vi "FeedbackDecode_UpdatePresetsTable.vi"(2 "StimClustIn":T1={"ParamsTable"=[], "Sel"=[], "Stim"=FALSE, "StimMode"=enum."Off", "StimStep"=[enum."1uA", enum."1uA", enum."Off"], "Jitter"=FALSE, "Pulse"=FALSE, "BFreq"=0.0, "BAmp"=0.0, "UEAArray"=[], "AdjClust"={"Add"=FALSE, "Sub"=FALSE, "Val"=[1.0, 100.0, 0.2, 500.0, 0.0], "B"=[FALSE, FALSE, FALSE, FALSE, FALSE], "Inc+"=["x+1", "x+10", "x+0.1", "x+10", "x+10"], "Set"=FALSE, "LoadTable"=FALSE, "SaveTable"=FALSE, "ClearTable"=FALSE, "DeleteSel"=FALSE, "Inc-"=["x-1", "x-10", "x-0.1", "x-10", "x-10"]}, "PresetTable"=[], "SelPreset"=[], "SortClust"={"Region"=FALSE, "Receptor"=FALSE, "Electrode"=FALSE, "Min Amp"=FALSE, "Max Amp"=FALSE, "Min Freq"=FALSE, "Max Freq"=FALSE, "Duration"=FALSE}, "SelSort"={"Sel"=FALSE}, "PresetClust"={"Load"=FALSE, "Clear"=FALSE, "Save"=FALSE, "Del"=FALSE}, "RespClust"={"RespType"=enum."Sensor Map", "OpenResp"=FALSE}, "AmpLimit"=0.0, "FreqLimit"=0.0, "DurLimit"=0.0, "Wait Period"=0.0, "Train Period"=0.0} {"Train Period" min=0.0 max=100.0 step=0.1; "Wait Period" min=0.0 max=100.0 step=0.1; "DurLimit" min=0.0 max=1.0 step=0.01; "FreqLimit" min=0.0 max=500.0 step=1.0; "AmpLimit" min=0.0 max=100.0 step=1.0; "BAmp" min=0.0 max=100.0 step=1.0; "BFreq" min=0.0 max=100.0 step=1.0}) -> (0 "StimClustOut":T1={"ParamsTable"=[], "Sel"=[], "Stim"=FALSE, "StimMode"=enum."Off", "StimStep"=[enum."1uA", enum."1uA", enum."Off"], "Jitter"=FALSE, "Pulse"=FALSE, "BFreq"=0.0, "BAmp"=0.0, "UEAArray"=[], "AdjClust"={"Add"=FALSE, "Sub"=FALSE, "Val"=[1.0, 100.0, 0.2, 500.0, 0.0], "B"=[FALSE, FALSE, FALSE, FALSE, FALSE], "Inc+"=["x+1", "x+10", "x+0.1", "x+10", "x+10"], "Set"=FALSE, "LoadTable"=FALSE, "SaveTable"=FALSE, "ClearTable"=FALSE, "DeleteSel"=FALSE, "Inc-"=["x-1", "x-10", "x-0.1", "x-10", "x-10"]}, "PresetTable"=[], "SelPreset"=[], "SortClust"={"Region"=FALSE, "Receptor"=FALSE, "Electrode"=FALSE, "Min Amp"=FALSE, "Max Amp"=FALSE, "Min Freq"=FALSE, "Max Freq"=FALSE, "Duration"=FALSE}, "SelSort"={"Sel"=FALSE}, "PresetClust"={"Load"=FALSE, "Clear"=FALSE, "Save"=FALSE, "Del"=FALSE}, "RespClust"={"RespType"=enum."Sensor Map", "OpenResp"=FALSE}, "AmpLimit"=0.0, "FreqLimit"=0.0, "DurLimit"=0.0, "Wait Period"=0.0, "Train Period"=0.0} {"Train Period" min=0.0 max=100.0 step=0.1; "Wait Period" min=0.0 max=100.0 step=0.1; "DurLimit" min=0.0 max=1.0 step=0.01; "FreqLimit" min=0.0 max=500.0 step=1.0; "AmpLimit" min=0.0 max=100.0 step=1.0; "BAmp" min=0.0 max=100.0 step=1.0; "BFreq" min=0.0 max=100.0 step=1.0})   [LabVIEW 2020]
uses:
  FeedbackDecode_EncodeClust.ctl
  <vilib>/regexp/Match Regular Expression.xnode
panel:
  # "Value"
  # "Inc-"
  # "Inc+"
  # "Min Amp"
  # "Max Amp"
  # "Min Freq"
  # "Max Freq"
  # "Duration"
  # "Value"
  # "Inc-"
  # "Inc+"
  # "Min Amp"
  # "Max Amp"
  # "Min Freq"
  # "Max Freq"
  # "Duration"
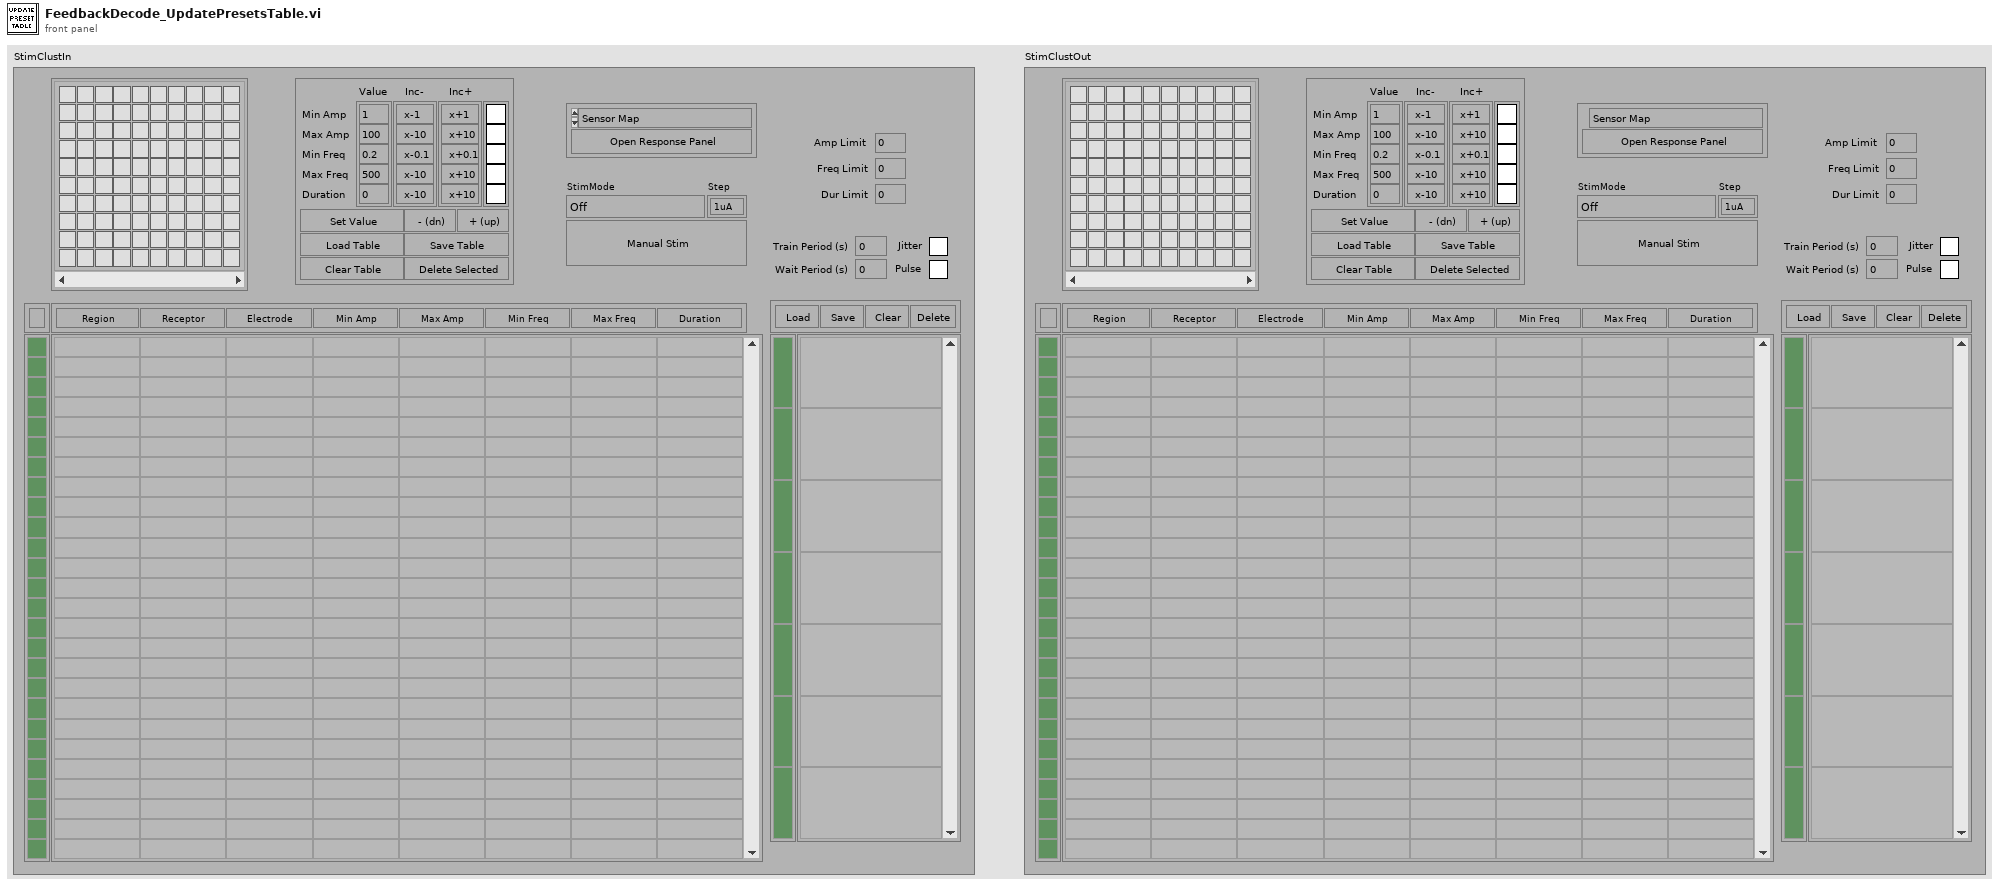
[diagram p1: front panel]
types:
  T1 = typedef "FeedbackDecode_EncodeClust.ctl" = cluster{"ParamsTable":string[][], "Sel":bool[], "Stim":bool, "StimMode":enum16{"Off", "Manual", "MSMS", "VRE", "3DHand", "DEKA", "Analog(DEKA)"}, "StimStep":enum16{"Off", "1uA", "2uA", "5uA", "10uA", "20uA", "30uA"}[], "Jitter":bool, "Pulse":bool, "BFreq":dbl, "BAmp":dbl, "UEAArray":cluster{"Boolean 1":bool, "Boolean 2":bool, "Boolean 3":bool, "Boolean 4":bool, "Boolean 5":bool, "Boolean 6":bool, "Boolean 7":bool, "Boolean 8":bool, "Boolean 9":bool, "Boolean 10":bool, "Boolean 11":bool, "Boolean 12":bool, "Boolean 13":bool, "Boolean 14":bool, "Boolean 15":bool, "Boolean 16":bool, "Boolean 17":bool, "Boolean 18":bool, "Boolean 19":bool, "Boolean 20":bool, "Boolean 21":bool, "Boolean 22":bool, "Boolean 23":bool, "Boolean 24":bool, "Boolean 25":bool, "Boolean 26":bool, "Boolean 27":bool, "Boolean 28":bool, "Boolean 29":bool, "Boolean 30":bool, "Boolean 31":bool, "Boolean 32":bool, "Boolean 33":bool, "Boolean 34":bool, "Boolean 35":bool, "Boolean 36":bool, "Boolean 37":bool, "Boolean 38":bool, "Boolean 39":bool, "Boolean 40":bool, "Boolean 41":bool, "Boolean 42":bool, "Boolean 43":bool, "Boolean 44":bool, "Boolean 45":bool, "Boolean 46":bool, "Boolean 47":bool, "Boolean 48":bool, "Boolean 49":bool, "Boolean 50":bool, "Boolean 51":bool, "Boolean 52":bool, "Boolean 53":bool, "Boolean 54":bool, "Boolean 55":bool, "Boolean 56":bool, "Boolean 57":bool, "Boolean 58":bool, "Boolean 59":bool, "Boolean 60":bool, "Boolean 61":bool, "Boolean 62":bool, "Boolean 63":bool, "Boolean 64":bool, "Boolean 65":bool, "Boolean 66":bool, "Boolean 67":bool, "Boolean 68":bool, "Boolean 69":bool, "Boolean 70":bool, "Boolean 71":bool, "Boolean 72":bool, "Boolean 73":bool, "Boolean 74":bool, "Boolean 75":bool, "Boolean 76":bool, "Boolean 77":bool, "Boolean 78":bool, "Boolean 79":bool, "Boolean 80":bool, "Boolean 81":bool, "Boolean 82":bool, "Boolean 83":bool, "Boolean 84":bool, "Boolean 85":bool, "Boolean 86":bool, "Boolean 87":bool, "Boolean 88":bool, "Boolean 89":bool, "Boolean 90":bool, "Boolean 91":bool, "Boolean 92":bool, "Boolean 93":bool, "Boolean 94":bool, "Boolean 95":bool, "Boolean 96":bool, "Boolean 97":bool, "Boolean 98":bool, "Boolean 99":bool, "Boolean 100":bool}[], "AdjClust":cluster{"Add":bool, "Sub":bool, "Val":dbl[], "B":bool[], "Inc+":string[], "Set":bool, "LoadTable":bool, "SaveTable":bool, "ClearTable":bool, "DeleteSel":bool, "Inc-":string[]}, "PresetTable":string[][], "SelPreset":bool[], "SortClust":cluster{"Region":bool, "Receptor":bool, "Electrode":bool, "Min Amp":bool, "Max Amp":bool, "Min Freq":bool, "Max Freq":bool, "Duration":bool}, "SelSort":cluster{"Sel":bool}, "PresetClust":cluster{"Load":bool, "Clear":bool, "Save":bool, "Del":bool}, "RespClust":cluster{"RespType":enum16{"Sensor Map", "Full Map"}, "OpenResp":bool}, "AmpLimit":dbl, "FreqLimit":dbl, "DurLimit":dbl, "Wait Period":dbl, "Train Period":dbl}
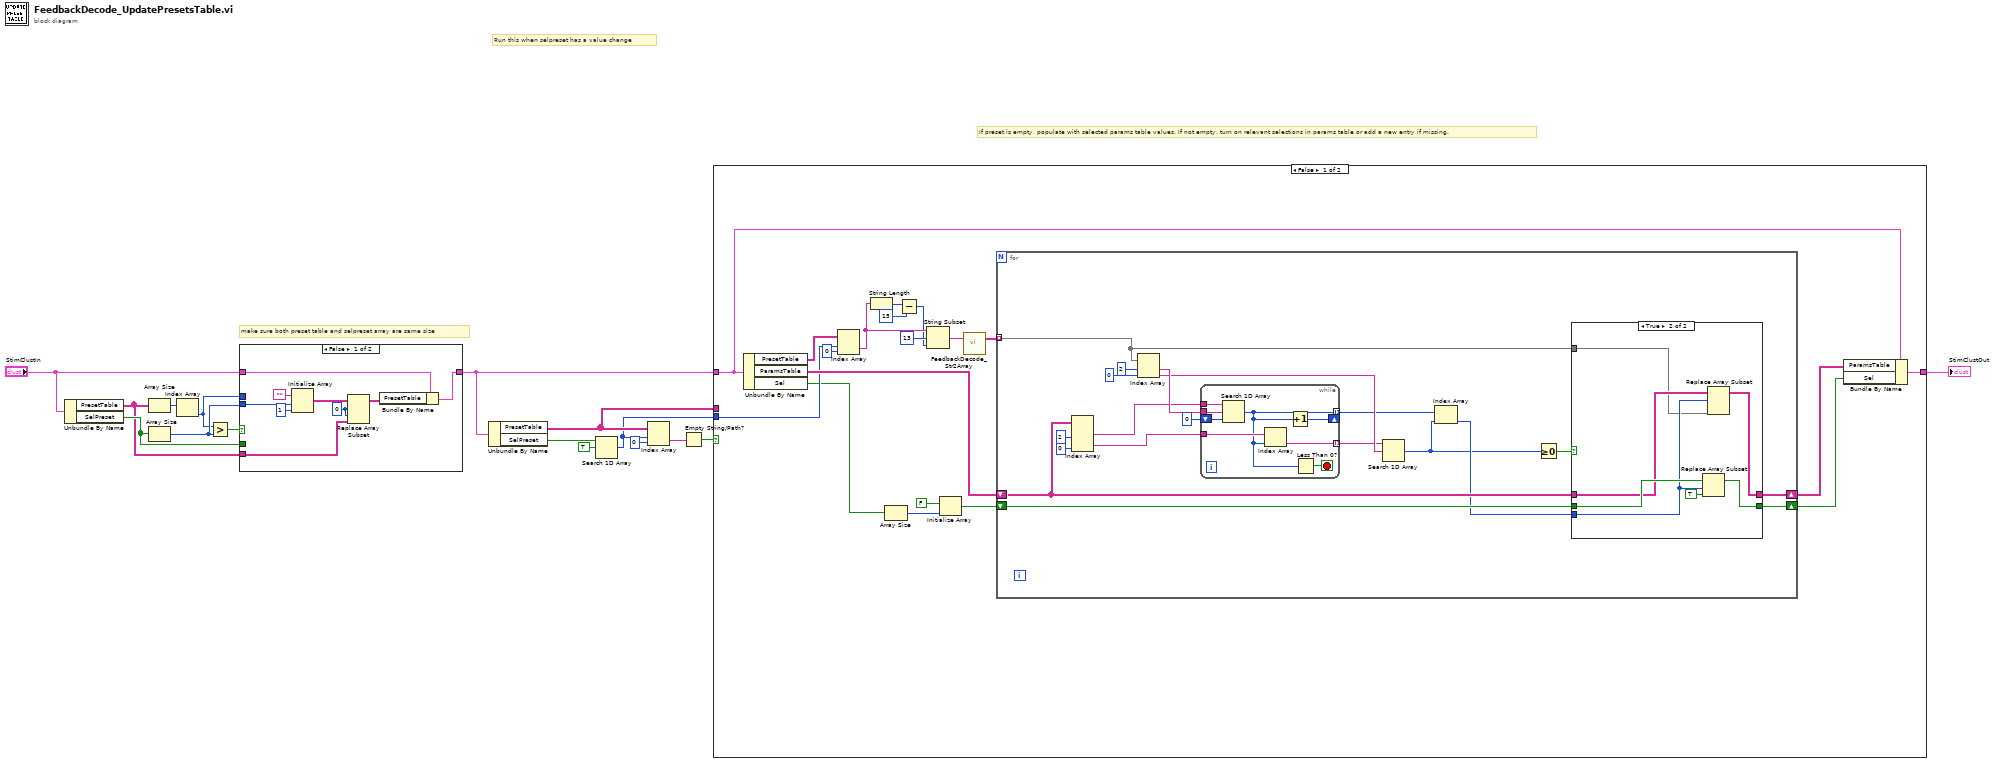
[diagram p0: block diagram]
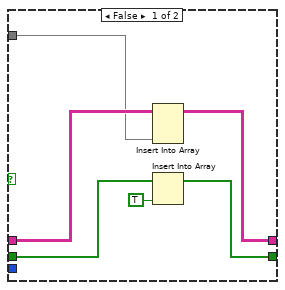
[diagram p2: hidden frame]
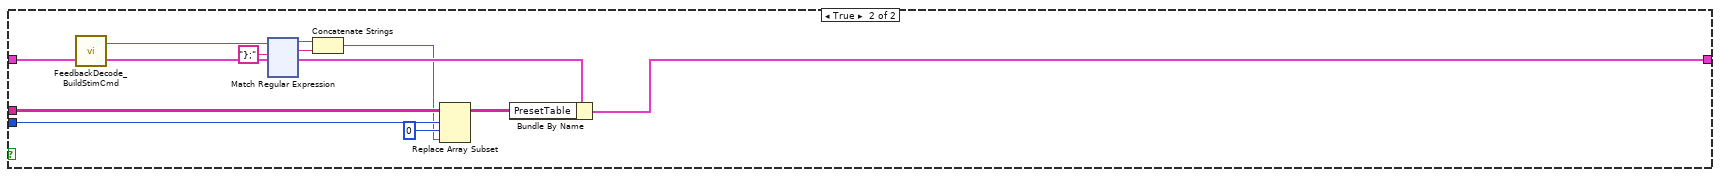
[diagram p3: hidden frame]
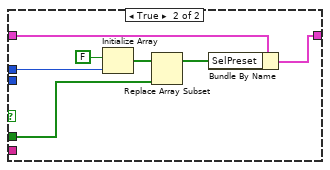
[diagram p4: hidden frame]
diagram:
  # "Run this when selpreset has a value change"
  # "If preset is empty, populate with selected params table values. If not empty, turn on relevant selections in params table or add a new entry if missing."
  # "make sure both preset table and selpreset array are same size"
  n1 = Unbundle By Name("StimClustIn") -> ("PresetTable"=w10:string[][], "SelPreset"=w14:bool[])
  n2 = Array Size(array=w10) -> (size(s)=w12:i32[])
  n3 = Array Size(array=w14) -> (size(s)=w16:i32)
  n4 = Index Array(array=w12) -> (element=w15:i32)  [unwired: 1 in]
  n5 = Greater?(x=w15, y=w16) -> (0:w13:bool)
  n6 = case shown="False" w13 {
    tunnel: "StimClustIn" -> [w23 w32]
    tunnel: [w22 w30] -> w4
    tunnel: w14 -> [_ w26]
    tunnel: w15 -> [_ w28]
    tunnel: w10 -> [w25 _]
    tunnel: w16 -> [w20 _]
    frame False {
      w24 = 0 ("index (row)")
      n7 = Initialize Array("", w20, 1 ("dimension size")) -> (w17:string[][])
      n8 = Replace Array Subset(array=w17, new element=w25, index (row)=w24, index (col)=w24) -> (w21:string[][])
      n9 = Bundle By Name(cluster=w23, "PresetTable"=w21) -> (w22:T1)
    }
    frame True {
      n10 = Initialize Array(FALSE ("new element/subarray"), w28) -> (w27:bool[])
      n11 = Replace Array Subset(array=w27, new element=w26) -> (w31:bool[])  [unwired: 1 in]
      n12 = Bundle By Name(cluster=w32, "SelPreset"=w31) -> (w30:T1)
    }
  }
  n13 = Unbundle By Name(w4) -> ("PresetTable"=w2:string[][], "SelPreset"=w9:bool[])
  n14 = Search 1D Array(1D array=w9, element=TRUE) -> (index of element=w1:i32)  [unwired: 1 in]
  n15 = Index Array(array=w2, index (row)=w1, index (col)=0 ("disabled index (col)")) -> (element=w7:string)
  n16 = Empty String/Path?(string/path=w7) -> (empty?=w6:bool)
  n17 = case shown="False" w6 {
    tunnel: w4 -> [w47 w97]
    tunnel: [w48 w98] -> w3
    tunnel: w2 -> [_ w102]
    tunnel: w1 -> [w45 w101]
    frame False {
      n18 = Unbundle By Name(w47) -> ("PresetTable"=w46:string[][], "ParamsTable"=w49:string[][], "Sel"=w37:bool[])
      n19 = Index Array(array=w46, index (row)=w45, index (col)=0 ("disabled index (col)")) -> (element=w40:string)
      n20 = String Length(string=w40) -> (length=w42:i32)
      n21 = Array Size(array=w37) -> (size(s)=w36:i32)
      n22 = Subtract(x=w42, y=15) -> (x-y=w38:i32)
      n23 = String Subset(string=w40, offset (0)=13, length (rest)=w38) -> (substring=w39:string)
      n24 = Initialize Array(FALSE, w36) -> (w34:bool[])
      n25 = call "FeedbackDecode_Str2Array.vi"("StringIn"=w39) -> ("StrArrayOut"=w33:string[][])  [unwired: 1 in, 1 out]
      n26 = for {
        shift-right: [w69] -> w51
        shift-left: w34 -> [w70]
        shift-right: [w67] -> w50
        shift-left: w49 -> [w68]
        tunnel: w33 -> [w53] mode=indexing
        n27 = Index Array(array=w68, index (col) #1=2 ("disabled index (col)"), index (col) #2=0 ("index (col)")) -> (element #1=w61:string[], element #2=w60:string[])  [unwired: 2 in]
        n28 = Index Array(array=w53, index #1=2 ("index"), index #2=0 ("index")) -> (element #1=w65:string, element #2=w59:string)
        n29 = while {
          tunnel: w61 -> [w78]
          tunnel: w65 -> [w77]
          shift-right: [w71] -> _
          shift-left: 0 ("disabled index (col)") -> [w76]
          tunnel: w60 -> [w75]
          tunnel: [w74] -> w58 mode=indexing
          tunnel: [w72] -> w57 mode=indexing
          stop <- w73 stop-if-true
          n30 = Search 1D Array(1D array=w78, element=w77, start index (0)=w76) -> (index of element=w72:i32)
          n31 = Index Array(array=w75, index=w72) -> (element=w74:string)
          n32 = Increment(x=w72) -> (x+1=w71:i32)
          n33 = Less Than 0?(x=w72) -> (x < 0?=w73:bool)
        }
        n34 = Search 1D Array(1D array=w58, element=w59) -> (index of element=w55:i32)  [unwired: 1 in]
        n35 = Index Array(array=w57, index=w55) -> (element=w56:i32)
        n36 = Greater Or Equal To 0?(x=w55) -> (x >= 0?=w54:bool)
        n37 = case shown="True" w54 {
          tunnel: w56 -> [_ w86]
          tunnel: w70 -> [w82 w91]
          tunnel: [w80 w89] -> w69
          tunnel: w68 -> [w84 w88]
          tunnel: [w83 w87] -> w67
          tunnel: w53 -> [w79 w85]
          frame False {
            n38 = Insert Into Array(array=w84, new element=w79) -> (w83:string[][])  [unwired: 2 in]
            n39 = Insert Into Array(array=w82, new element=TRUE ("new element/subarray")) -> (w80:bool[])  [unwired: 1 in]
          }
          frame True {
            n40 = Replace Array Subset(array=w91, new element=TRUE ("new element/subarray"), index=w86) -> (w89:bool[])
            n41 = Replace Array Subset(array=w88, new element=w85, index (row)=w86) -> (w87:string[][])  [unwired: 1 in]
          }
        }
      }
      n42 = Bundle By Name(cluster=w47, "ParamsTable"=w50, "Sel"=w51) -> (w48:T1)
    }
    frame True {
      n43 = call "FeedbackDecode_BuildStimCmd.vi"("EncodeClustIn"=w97) -> ("EncodeClustOut"=w103:T1, "StimCmd"=w96:string)  [unwired: 1 in]
      n44 = xnode "Match Regular Expression"("input string"=w96, "regular expression"="};") -> ("before match"=w94:string, "whole match"=w93:string)  [unwired: 4 in, 3 out]
      n45 = Concatenate Strings(w94, w93) -> (w92:string)
      n46 = Replace Array Subset(array=w102, new element=w92, index (row)=w101, index (col)=0 ("disabled index (col)")) -> (w99:string[][])
      n47 = Bundle By Name(cluster=w103, "PresetTable"=w99) -> (w98:T1)
    }
  }
  "StimClustOut" <- w3
